vi "xiUtils - Check if File or Folder exists.vi"(8 "error in (no error)":errorcluster, 11 "path":path) -> (0 "error out":errorcluster, 2 "file or folder exists?":bool, 3 "dup path":path)   [LabVIEW 2018]
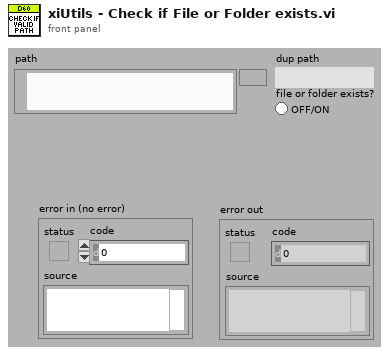
[diagram p1: front panel]
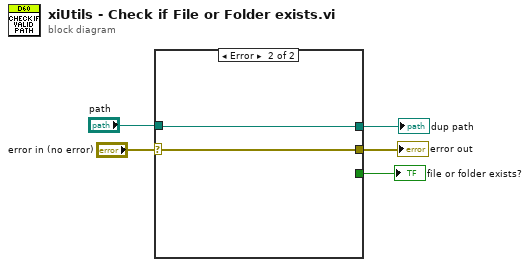
[diagram p0: block diagram]
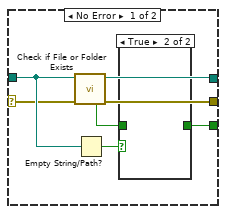
[diagram p2: hidden frame]
diagram:
  n1 = case shown="Error" "error in (no error)" {
    selector: "error in (no error)" -> [w11 w14]
    tunnel: "path" -> [w12 w15]
    tunnel: [w10 w15] -> w3
    tunnel: [w9 w14] -> w2
    tunnel: [w6 _] -> w1
    frame No Error {
      n2 = call <vilib>:"Check if File or Folder Exists.vi"("error in (no error)"=w11, "path"=w12) -> ("error out"=w9:errorcluster, "file or folder exists?"=w7:bool, "dup path"=w10:path)  [unwired: 7 in]
      n3 = Empty String/Path?(string/path=w12) -> (empty?=w8:bool)
      n4 = case shown="True" w8 {
        tunnel: w7 -> [w13 _]
        tunnel: [w13 _] -> w6
        frame False {
        }
        frame True {
        }
      }
    }
    frame Error {
    }
  }
  "error out" <- w2
  "dup path" <- w3
  "file or folder exists?" <- w1
